vi "0037-Sub_graph2.vi"(6 "グラフプロット数":i32, 7 "温湿度データ":dbl[][](array[numeric])) -> (1 "温度":T1, 3 "湿度":T1)   [LabVIEW 2014]
panel:
  out "2":dbl[][](array[numeric])
  out "1":dbl[][](array[numeric])
  out "3":dbl[][](array[numeric])
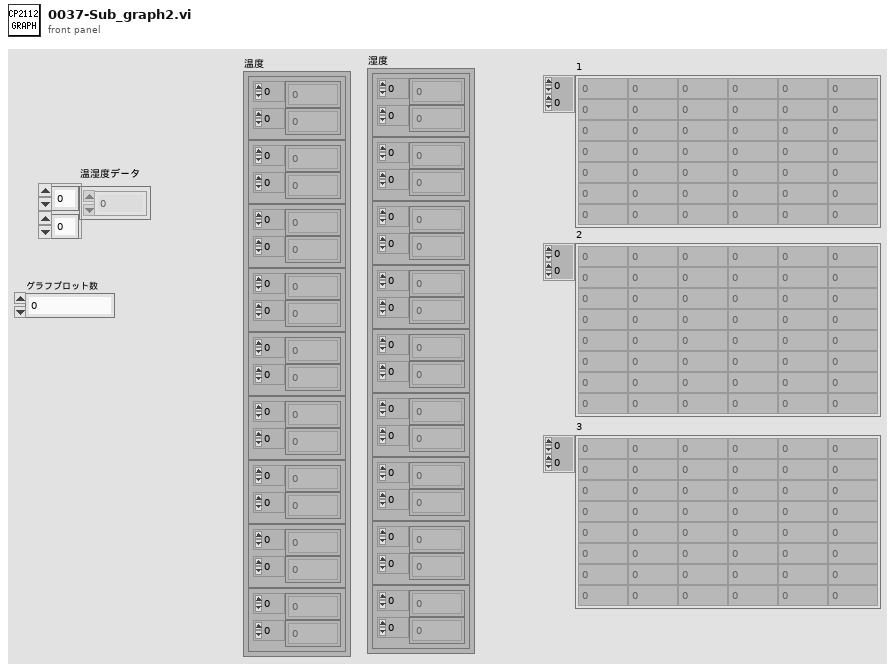
[diagram p1: front panel]
types:
  T1 = cluster{cluster{dbl[], dbl[]}, cluster{dbl[], dbl[]}, cluster{dbl[], dbl[]}, cluster{dbl[], dbl[]}, cluster{dbl[], dbl[]}, cluster{dbl[], dbl[]}, cluster{dbl[], dbl[]}, cluster{dbl[], dbl[]}, cluster{dbl[], dbl[]}}
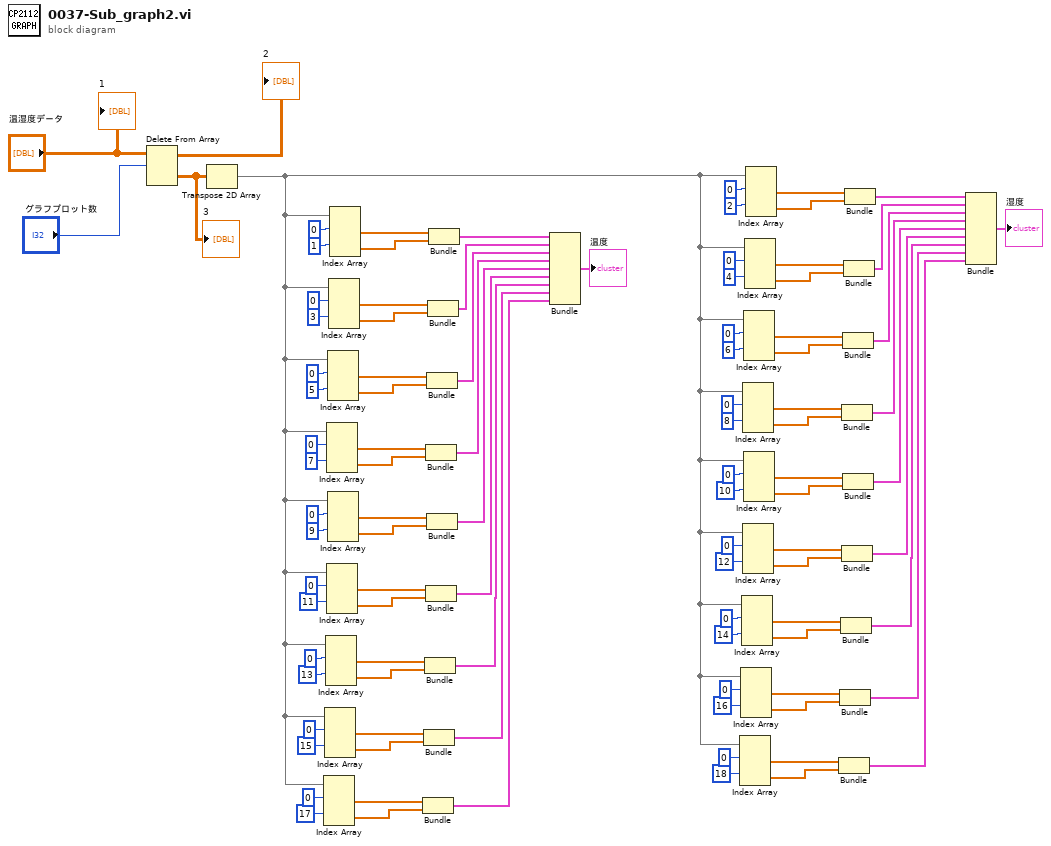
[diagram p0: block diagram]
diagram:
  n1 = Delete From Array(array="温湿度データ", length="グラフプロット数") -> (deleted portion=w1:dbl[][], array with subset deleted=→"2":dbl[][])  [unwired: 2 in]
  "3" <- w1
  n2 = Transpose 2D Array(2D array=w1) -> (transposed array=w2:dbl[][])
  n3 = Index Array(array=w2, index (row) #1=0 ("指標 （行）"), index (row) #2=17 ("指標 （行）")) -> (element #1=w61:dbl[], element #2=w60:dbl[])  [unwired: 2 in]
  n4 = Index Array(array=w2, index (row) #1=0 ("指標 （行）"), index (row) #2=15 ("指標 （行）")) -> (element #1=w65:dbl[], element #2=w64:dbl[])  [unwired: 2 in]
  n5 = Index Array(array=w2, index (row) #1=0 ("指標 （行）"), index (row) #2=13 ("指標 （行）")) -> (element #1=w69:dbl[], element #2=w68:dbl[])  [unwired: 2 in]
  n6 = Index Array(array=w2, index (row) #1=0 ("指標 （行）"), index (row) #2=7 ("指標 （行）")) -> (element #1=w81:dbl[], element #2=w80:dbl[])  [unwired: 2 in]
  n7 = Index Array(array=w2, index (row) #1=0 ("指標 （行）"), index (row) #2=11 ("指標 （行）")) -> (element #1=w73:dbl[], element #2=w72:dbl[])  [unwired: 2 in]
  n8 = Index Array(array=w2, index (row) #1=0 ("指標 （行）"), index (row) #2=5 ("指標 （行）")) -> (element #1=w85:dbl[], element #2=w84:dbl[])  [unwired: 2 in]
  n9 = Index Array(array=w2, index (row) #1=0 ("指標 （行）"), index (row) #2=9 ("指標 （行）")) -> (element #1=w77:dbl[], element #2=w76:dbl[])  [unwired: 2 in]
  n10 = Index Array(array=w2, index (row) #1=0 ("指標 （行）"), index (row) #2=3 ("指標 （行）")) -> (element #1=w91:dbl[], element #2=w90:dbl[])  [unwired: 2 in]
  n11 = Index Array(array=w2, index (row) #1=0 ("指標 （行）"), index (row) #2=1 ("指標 （行）")) -> (element #1=w95:dbl[], element #2=w94:dbl[])  [unwired: 2 in]
  n12 = Bundle(w61, w60) -> (w53:cluster{dbl[], dbl[]})  [unwired: 1 in]
  n13 = Bundle(w65, w64) -> (w54:cluster{dbl[], dbl[]})  [unwired: 1 in]
  n14 = Bundle(w69, w68) -> (w55:cluster{dbl[], dbl[]})  [unwired: 1 in]
  n15 = Bundle(w81, w80) -> (w58:cluster{dbl[], dbl[]})  [unwired: 1 in]
  n16 = Bundle(w73, w72) -> (w56:cluster{dbl[], dbl[]})  [unwired: 1 in]
  n17 = Bundle(w85, w84) -> (w59:cluster{dbl[], dbl[]})  [unwired: 1 in]
  n18 = Bundle(w77, w76) -> (w57:cluster{dbl[], dbl[]})  [unwired: 1 in]
  n19 = Bundle(w91, w90) -> (w88:cluster{dbl[], dbl[]})  [unwired: 1 in]
  n20 = Bundle(w95, w94) -> (w89:cluster{dbl[], dbl[]})  [unwired: 1 in]
  n21 = Bundle(w89, w88, w59, w58, w57, w56, w55, w54, w53) -> (→"温度":T1)  [unwired: 1 in]
  n22 = Index Array(array=w2, index (row) #1=0 ("指標 （行）"), index (row) #2=18 ("指標 （行）")) -> (element #1=w15:dbl[], element #2=w14:dbl[])  [unwired: 2 in]
  n23 = Index Array(array=w2, index (row) #1=0 ("指標 （行）"), index (row) #2=16 ("指標 （行）")) -> (element #1=w19:dbl[], element #2=w18:dbl[])  [unwired: 2 in]
  n24 = Index Array(array=w2, index (row) #1=0 ("指標 （行）"), index (row) #2=14 ("指標 （行）")) -> (element #1=w23:dbl[], element #2=w22:dbl[])  [unwired: 2 in]
  n25 = Index Array(array=w2, index (row) #1=0 ("指標 （行）"), index (row) #2=8 ("指標 （行）")) -> (element #1=w35:dbl[], element #2=w34:dbl[])  [unwired: 2 in]
  n26 = Index Array(array=w2, index (row) #1=0 ("指標 （行）"), index (row) #2=12 ("指標 （行）")) -> (element #1=w27:dbl[], element #2=w26:dbl[])  [unwired: 2 in]
  n27 = Index Array(array=w2, index (row) #1=0 ("指標 （行）"), index (row) #2=6 ("指標 （行）")) -> (element #1=w39:dbl[], element #2=w38:dbl[])  [unwired: 2 in]
  n28 = Index Array(array=w2, index (row) #1=0 ("指標 （行）"), index (row) #2=10 ("指標 （行）")) -> (element #1=w31:dbl[], element #2=w30:dbl[])  [unwired: 2 in]
  n29 = Index Array(array=w2, index (row) #1=0 ("指標 （行）"), index (row) #2=4 ("指標 （行）")) -> (element #1=w45:dbl[], element #2=w44:dbl[])  [unwired: 2 in]
  n30 = Index Array(array=w2, index (row) #1=0 ("指標 （行）"), index (row) #2=2 ("指標 （行）")) -> (element #1=w49:dbl[], element #2=w48:dbl[])  [unwired: 2 in]
  n31 = Bundle(w15, w14) -> (w7:cluster{dbl[], dbl[]})  [unwired: 1 in]
  n32 = Bundle(w19, w18) -> (w8:cluster{dbl[], dbl[]})  [unwired: 1 in]
  n33 = Bundle(w23, w22) -> (w9:cluster{dbl[], dbl[]})  [unwired: 1 in]
  n34 = Bundle(w35, w34) -> (w12:cluster{dbl[], dbl[]})  [unwired: 1 in]
  n35 = Bundle(w27, w26) -> (w10:cluster{dbl[], dbl[]})  [unwired: 1 in]
  n36 = Bundle(w39, w38) -> (w13:cluster{dbl[], dbl[]})  [unwired: 1 in]
  n37 = Bundle(w31, w30) -> (w11:cluster{dbl[], dbl[]})  [unwired: 1 in]
  n38 = Bundle(w45, w44) -> (w42:cluster{dbl[], dbl[]})  [unwired: 1 in]
  n39 = Bundle(w49, w48) -> (w43:cluster{dbl[], dbl[]})  [unwired: 1 in]
  n40 = Bundle(w43, w42, w13, w12, w11, w10, w9, w8, w7) -> (→"湿度":T1)  [unwired: 1 in]
  "1" <- "温湿度データ"
